vi "Refresh References.vi"(8 "error in (no error)":errorcluster, 11 "CSM-Helper in":refnum<class "CSM-Helper.lvclass">) -> (0 "error out":errorcluster, 3 "CSM-Helper out":refnum<class "CSM-Helper.lvclass">)   [LabVIEW 2017, in "CSM-Helper.lvclass"]
doc: "### Refresh References.vi\n\n-- <b>Controls</b> --\n- <b>CSM-Helper in</b>: CSMHelper input\n\n-- <b>Indicators</b> --\n- <b>CSM-Helper out</b>: CSMHelper output"
uses:
  CSM-Helper.lvclass
  CSM-Helper.lvclass/CSM-Helper.ctl
  <vilib>/Utility/Data Type/Type Definitions/Data Type.ctl
  <vilib>/Utility/Data Type/Type Definitions/Refnum Type.ctl
  <vilib>/Utility/Data Type/NI_Data Type.lvlib
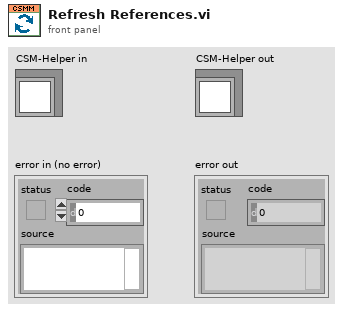
[diagram p1: front panel]
types:
  T1 = typedef "NI_Data Type.lvlib/Refnum Type.ctl" = enum16{"NotARefnum", "UnknownRefnum", "Generic", "Datalog", "ByteStream", "Device", "Occurence", "TCPNetConnection", "Auto", "Menu", "Imaq", "Hardware", "DataSocket", "Visa", "IVI", "UDPNetConnection", "Notifier", "Queue", "Irda", "EventReg", "DotNet", "UserEvent", "Callback", "UNUSED_EMPTY_POSITION", "BlueToothNetConnection", "LVObjApp", "LVObjVI", "LVObjUnknown", "GenericClass", "UserDefinedRefnumTag", "DataValue", "RT FIFO", "TDMS File"}
  T2 = typedef "NI_Data Type.lvlib/Data Type.ctl" = enum8{"Invalid Type", "Void", "I8", "I16", "I32", "I64", "U8", "U16", "U32", "U64", "Single Float", "Double Float", "Extended Float", "Single Complex", "Double Complex", "Extended Complex", "Enum U8", "Enum U16", "Enum U32", "Enum U64", "Single Float With Unit", "Double Float With Unit", "Extended Float With Unit", "Single Complex with Unit", "Double Complex with Unit", "Extended Complex with Unit", "Boolean", "String", "Path", "Picture", "Tag", "Array", "Cluster", "Variant", "LV Variant", "Waveform", "Timestamp", "Digital Waveform", "Digital Data", "ExpressData", "Refnum", "External Data", "VI", "Poly VI", "LabVIEW Class Instance", "Fixed Point"}
  T3 = cluster{refnum<vi>, "Outer Term":refnum<vi>, "Data Type":variant, "Wire":refnum<vi>}
  T4 = typedef "NI_Data Type.lvlib/Type Definition Info.ctl" = cluster{"Name":string, "Timestamp":u32}
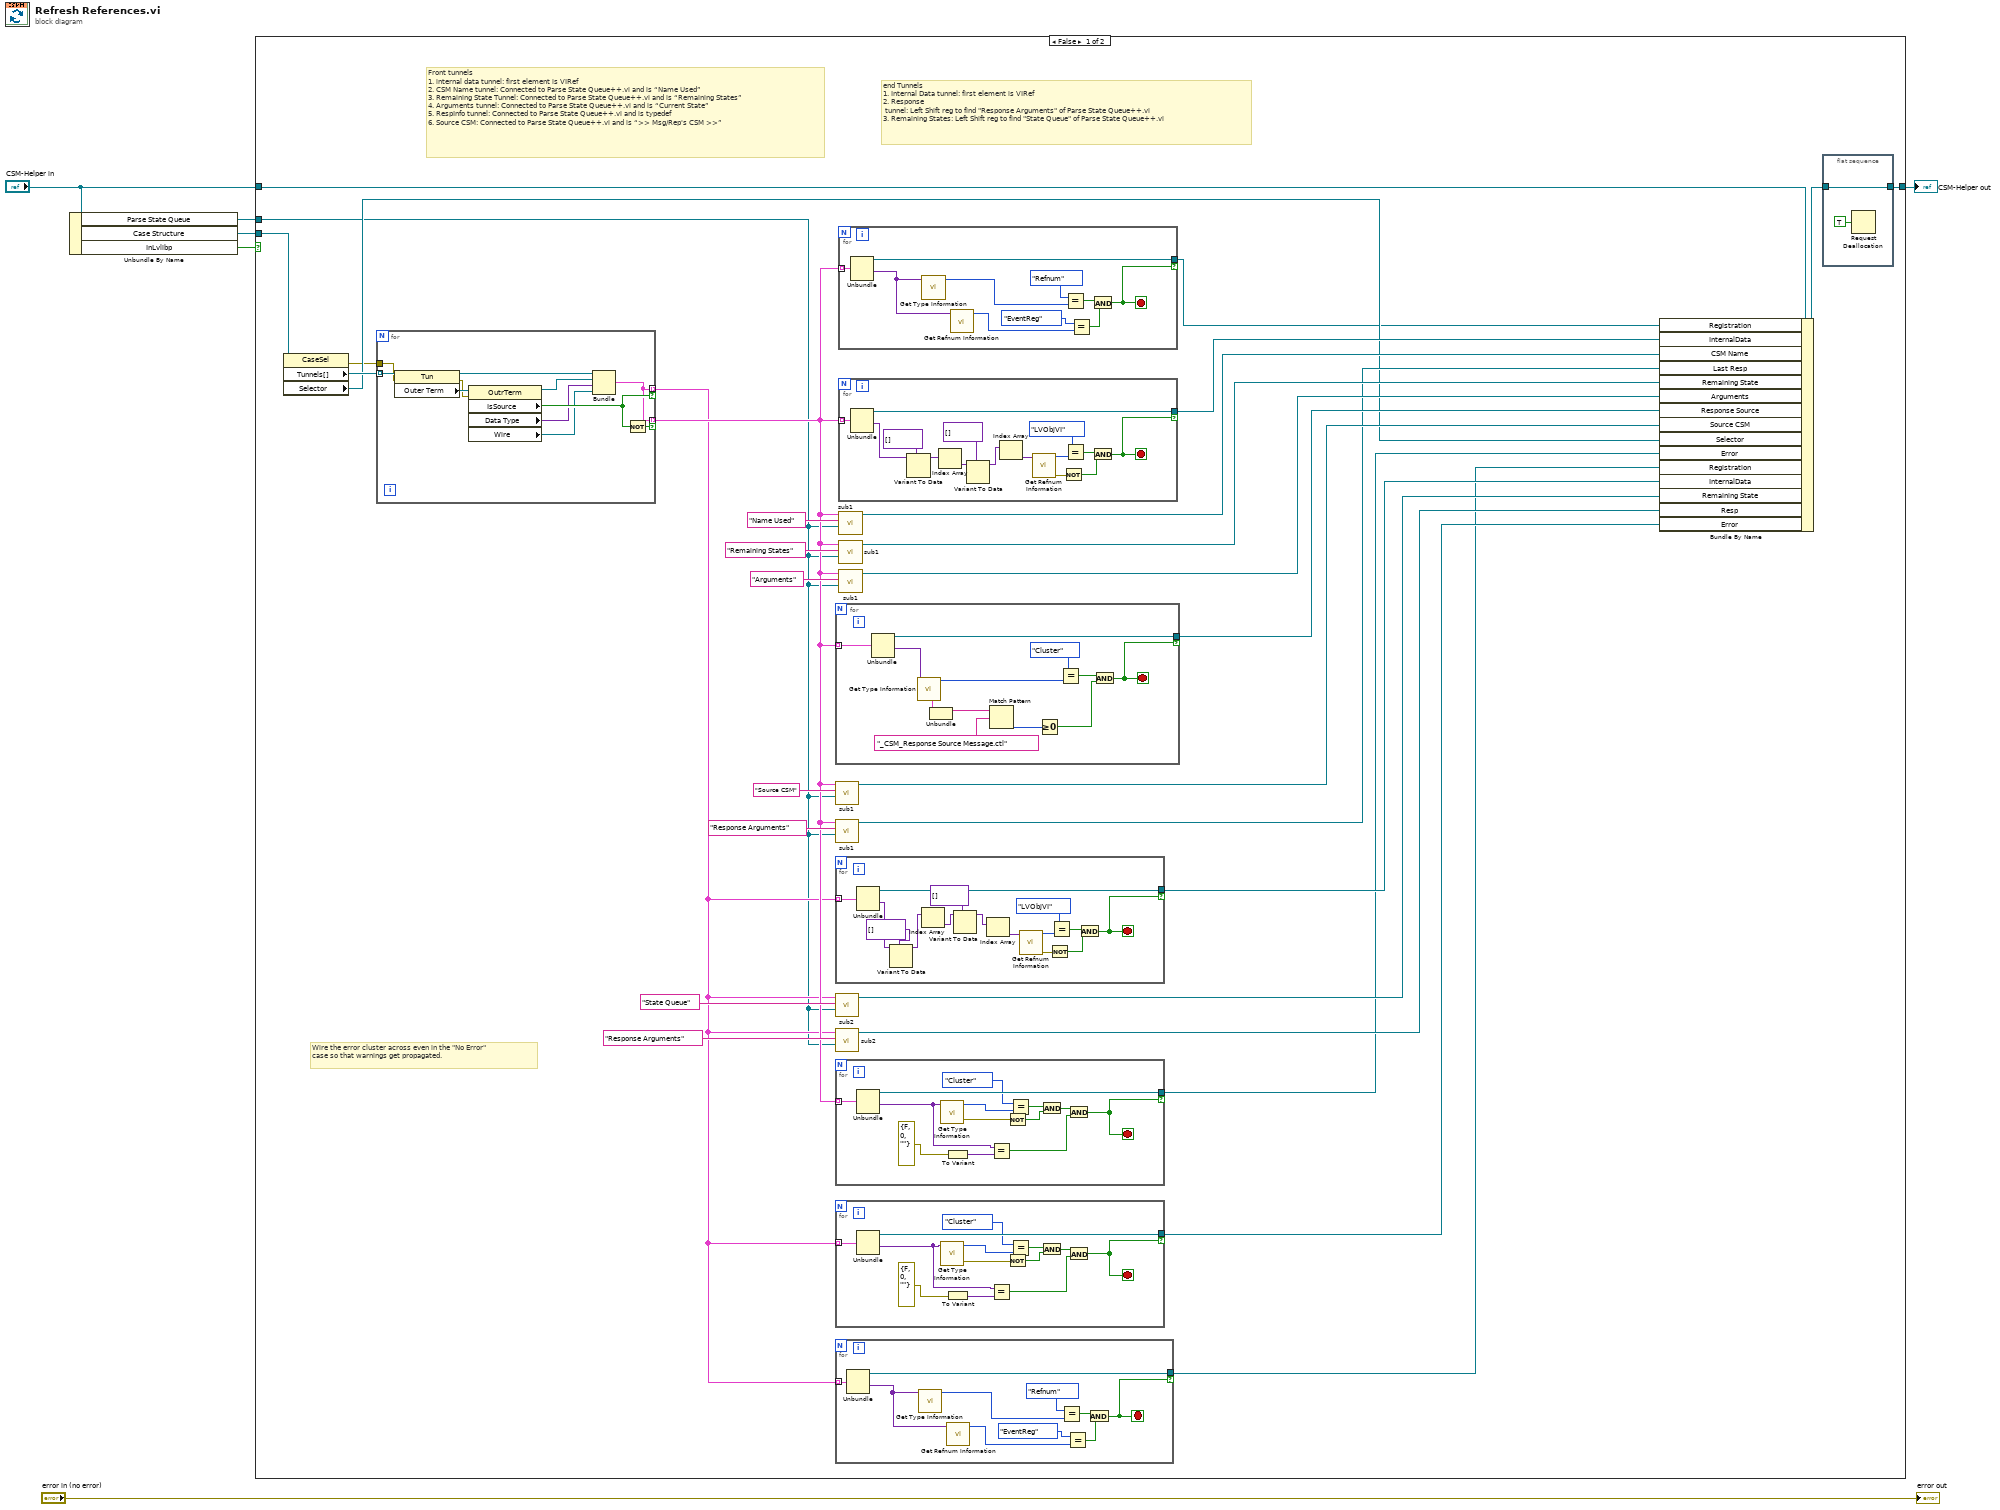
[diagram p0: block diagram]
diagram:
  n1 = Unbundle By Name("CSM-Helper in") -> ("Parse State Queue"=w2:refnum<vi>, "Case Structure"=w4:refnum<vi>, "InLvlibp"=w1:bool)
  n2 = case shown="False" w1 {
    tunnel: "CSM-Helper in" -> [w37 w139]
    tunnel: w4 -> [w36 _]
    tunnel: [w20 w139] -> w3
    tunnel: w2 -> [w8 _]
    frame False {
      # "end Tunnels\n1. Internal Data tunnel: first element is VIRef\n2. Response\n tunnel: Left Shift reg to find \"Response Arguments\" of Parse State Queue++.vi \n3. Remaining States: Left Shift reg to find \"State Queue\" of Parse State Queue++.vi"
      # "Front tunnels\n1. internal data tunnel: first element is VIRef\n2. CSM Name tunnel: Connected to Parse State Queue++.vi and is “Name Used”\n3. Remaining State Tunnel: Connected to Parse State Queue++.vi and is “Remaining States”\n4. Arguments tunnel: Connected to Parse State Queue++.vi and is “Current State”\n5. RespInfo tunnel: Connected to Parse State Queue++.vi and is typedef\n6. Source CSM: Connected to Parse State Queue++.vi and is “>> Msg/Rep's CSM >>”"
      # "Wire the error cluster across even in the \"No Error\"\ncase so that warnings get propagated."
      n3 = property class="CaseSel"(reference=w36) -> (error out=w7:errorcluster, "Tunnels[]"=w35:refnum<vi>[], "Selector"=w22:refnum<vi>)  [unwired: 1 in, 1 out]
      n4 = for {
        tunnel: w35 -> [w111] mode=indexing
        tunnel: [w104] -> w10 mode=indexing if=w108
        tunnel: [w104] -> w12 mode=indexing if=w107
        tunnel: w7 -> [w101]
        n5 = property class="Tun"(reference=w111, error in=w101) -> (reference out=w106:refnum<vi>, error out=w109:errorcluster, "Outer Term"=w110:refnum<vi>)
        n6 = property class="OutrTerm"(reference=w110, error in=w109) -> (reference out=w105:refnum<vi>, "IsSource"=w108:bool, "Data Type"=w103:variant, "Wire"=w102:refnum<vi>)  [unwired: 1 out]
        n7 = Bundle(w106, "Outer Term"=w105, "Data Type"=w103, "Wire"=w102) -> (w104:T3)  [unwired: 1 in]
        n8 = Not(x=w108) -> (.not. x?=w107:bool)
      }
      n9 = for {
        tunnel: w12 -> [w123] mode=indexing
        tunnel: [w120] -> w25 if=w119
        stop <- w119 stop-if-true
        n10 = Unbundle(w123) -> (w120:refnum<vi>, "Data Type"=w116:variant)  [unwired: 2 out]
        n11 = call <vilib>:"Get Type Information.vi"("Variant"=w116) -> ("Type"=w122:T2, "Type Definition Info"=w117:T4)  [unwired: 6 in, 3 out]
        n12 = Unbundle(w117) -> ("Name"=w115:string)  [unwired: 1 out]
        n13 = Match Pattern(string=w115, regular expression="_CSM_Response Source Message.ctl") -> (offset past match=w113:i32)  [unwired: 1 in, 3 out]
        n14 = Greater Or Equal To 0?(x=w113) -> (x >= 0?=w112:bool)
        n15 = Equal?(x=Data_Type."Cluster", y=w122) -> (x = y?=w121:bool)
        n16 = And(x=w121, y=w112) -> (x .and. y?=w119:bool)
      }
      n17 = call "sub1.vi"("Part References.Parse State Queue"=w8, "regular expression"="Source CSM", "Array"=w12) -> ("Tunnel out"=w26:refnum<vi>)  [unwired: 8 in]
      n18 = call "sub1.vi"("Part References.Parse State Queue"=w8, "regular expression"="Response Arguments", "Array"=w12) -> ("Tunnel out"=w23:refnum<vi>)  [unwired: 8 in]
      n19 = for {
        tunnel: w10 -> [w100] mode=indexing
        tunnel: [w93] -> w19 if=w92
        stop <- w92 stop-if-true
        n20 = Unbundle(w100) -> (w93:refnum<vi>, "Data Type"=w88:variant)  [unwired: 2 out]
        n21 = Variant To Data(type=variant[] [] ("Array"), Variant=w88) -> (data=w86:variant[])  [unwired: 1 in, 1 out]
        n22 = Index Array(array=w86) -> (element=w90:variant)  [unwired: 1 in]
        n23 = Variant To Data(type=variant[] [] ("Array"), Variant=w90) -> (data=w89:variant[])  [unwired: 1 in, 1 out]
        n24 = Index Array(array=w89) -> (element=w99:variant)  [unwired: 1 in]
        n25 = call <vilib>:"Get Refnum Information.vi"("Variant"=w99) -> ("error out"=w95:errorcluster, "Reference Type"=w97:T1)  [unwired: 7 in, 2 out]
        n26 = Not(x=w95) -> (.not. x?=w94:bool)
        n27 = Equal?(x=Refnum_Type."LVObjVI", y=w97) -> (x = y?=w96:bool)
        n28 = And(x=w96, y=w94) -> (x .and. y?=w92:bool)
      }
      n29 = call "sub2.vi"("Part References.Parse State Queue"=w8, "regular expression"="State Queue", "Array"=w10) -> ("Tunnel out"=w17:refnum<vi>)  [unwired: 8 in]
      n30 = call "sub2.vi"("Part References.Parse State Queue"=w8, "regular expression"="Response Arguments", "Array"=w10) -> ("Tunnel out"=w15:refnum<vi>)  [unwired: 8 in]
      n31 = for {
        tunnel: w12 -> [w60] mode=indexing
        tunnel: [w59] -> w14 if=w48
        stop <- w48 stop-if-true
        n32 = Unbundle(w60) -> (w59:refnum<vi>, "Data Type"=w55:variant)  [unwired: 2 out]
        n33 = call <vilib>:"Get Type Information.vi"("Variant"=w55) -> ("error out"=w56:errorcluster, "Type"=w58:T2)  [unwired: 6 in, 3 out]
        n34 = To Variant(anything=errorcluster {"status"=FALSE, "code"=0, "source"=""} ("error in (no error)")) -> (Variant=w53:variant)
        n35 = Equal?(x=w55, y=w53) -> (x = y?=w49:bool)
        n36 = Not(x=w56) -> (.not. x?=w51:bool)
        n37 = Equal?(x=Data_Type."Cluster", y=w58) -> (x = y?=w52:bool)
        n38 = And(x=w52, y=w51) -> (x .and. y?=w50:bool)
        n39 = And(x=w50, y=w49) -> (x .and. y?=w48:bool)
      }
      n40 = for {
        tunnel: w10 -> [w73] mode=indexing
        tunnel: [w72] -> w13 if=w61
        stop <- w61 stop-if-true
        n41 = Unbundle(w73) -> (w72:refnum<vi>, "Data Type"=w68:variant)  [unwired: 2 out]
        n42 = call <vilib>:"Get Type Information.vi"("Variant"=w68) -> ("error out"=w69:errorcluster, "Type"=w71:T2)  [unwired: 6 in, 3 out]
        n43 = To Variant(anything=errorcluster {"status"=FALSE, "code"=0, "source"=""} ("error in (no error)")) -> (Variant=w66:variant)
        n44 = Equal?(x=w68, y=w66) -> (x = y?=w62:bool)
        n45 = Not(x=w69) -> (.not. x?=w64:bool)
        n46 = Equal?(x=Data_Type."Cluster", y=w71) -> (x = y?=w65:bool)
        n47 = And(x=w65, y=w64) -> (x .and. y?=w63:bool)
        n48 = And(x=w63, y=w62) -> (x .and. y?=w61:bool)
      }
      n49 = for {
        tunnel: w10 -> [w47] mode=indexing
        tunnel: [w45] -> w9 if=w44
        stop <- w44 stop-if-true
        n50 = Unbundle(w47) -> (w45:refnum<vi>, "Data Type"=w43:variant)  [unwired: 2 out]
        n51 = call <vilib>:"Get Type Information.vi"("Variant"=w43) -> ("Type"=w42:T2)  [unwired: 6 in, 4 out]
        n52 = call <vilib>:"Get Refnum Information.vi"("Variant"=w43) -> ("Reference Type"=w39:T1)  [unwired: 7 in, 3 out]
        n53 = Equal?(x=Data_Type."Refnum", y=w42) -> (x = y?=w46:bool)
        n54 = Equal?(x=Refnum_Type."EventReg" ("Reference Type"), y=w39) -> (x = y?=w38:bool)
        n55 = And(x=w46, y=w38) -> (x .and. y?=w44:bool)
      }
      n56 = for {
        tunnel: w12 -> [w85] mode=indexing
        tunnel: [w83] -> w11 if=w82
        stop <- w82 stop-if-true
        n57 = Unbundle(w85) -> (w83:refnum<vi>, "Data Type"=w81:variant)  [unwired: 2 out]
        n58 = call <vilib>:"Get Type Information.vi"("Variant"=w81) -> ("Type"=w80:T2)  [unwired: 6 in, 4 out]
        n59 = call <vilib>:"Get Refnum Information.vi"("Variant"=w81) -> ("Reference Type"=w77:T1)  [unwired: 7 in, 3 out]
        n60 = Equal?(x=Data_Type."Refnum", y=w80) -> (x = y?=w84:bool)
        n61 = Equal?(x=Refnum_Type."EventReg" ("Reference Type"), y=w77) -> (x = y?=w76:bool)
        n62 = And(x=w84, y=w76) -> (x .and. y?=w82:bool)
      }
      n63 = for {
        tunnel: w12 -> [w138] mode=indexing
        tunnel: [w131] -> w34 if=w130
        stop <- w130 stop-if-true
        n64 = Unbundle(w138) -> (w131:refnum<vi>, "Data Type"=w128:variant)  [unwired: 2 out]
        n65 = Variant To Data(type=variant[] [] ("Array"), Variant=w128) -> (data=w127:variant[])  [unwired: 1 in, 1 out]
        n66 = Index Array(array=w127) -> (element=w125:variant)  [unwired: 1 in]
        n67 = Variant To Data(type=variant[] [] ("Array"), Variant=w125) -> (data=w124:variant[])  [unwired: 1 in, 1 out]
        n68 = Index Array(array=w124) -> (element=w137:variant)  [unwired: 1 in]
        n69 = call <vilib>:"Get Refnum Information.vi"("Variant"=w137) -> ("error out"=w133:errorcluster, "Reference Type"=w135:T1)  [unwired: 7 in, 2 out]
        n70 = Not(x=w133) -> (.not. x?=w132:bool)
        n71 = Equal?(x=Refnum_Type."LVObjVI", y=w135) -> (x = y?=w134:bool)
        n72 = And(x=w134, y=w132) -> (x .and. y?=w130:bool)
      }
      n73 = call "sub1.vi"("Part References.Parse State Queue"=w8, "regular expression"="Name Used", "Array"=w12) -> ("Tunnel out"=w33:refnum<vi>)  [unwired: 8 in]
      n74 = call "sub1.vi"("Part References.Parse State Queue"=w8, "regular expression"="Remaining States", "Array"=w12) -> ("Tunnel out"=w30:refnum<vi>)  [unwired: 8 in]
      n75 = call "sub1.vi"("Part References.Parse State Queue"=w8, "regular expression"="Arguments", "Array"=w12) -> ("Tunnel out"=w28:refnum<vi>)  [unwired: 8 in]
      n76 = Bundle By Name(cluster=w37, "Registration"=w11, "InternalData"=w34, "CSM Name"=w33, "Last Resp"=w23, "Remaining State"=w30, "Arguments"=w28, "Response Source"=w25, "Source CSM"=w26, "Selector"=w22, "Error"=w14, "Registration"=w9, "InternalData"=w19, "Remaining State"=w17, "Resp"=w15, "Error"=w13) -> (w21:refnum<class "CSM-Helper.lvclass">)
      n77 = flat-sequence {
        tunnel: w21 -> [w74]
        tunnel: [w74] -> w20
        frame #0 {
          n78 = Request Deallocation(TRUE ("flag")) -> ()
        }
      }
    }
    frame True {
    }
  }
  "CSM-Helper out" <- w3
  "error out" <- "error in (no error)"
